vi "salRegSubEventsView.vi"(8 "error in (no error)":errorcluster, 11 "MiddlewareSALThisComponent in":refnum<class "MiddlewareSALThisComponent.lvclass">) -> (0 "error out":errorcluster, 2 "Event Registration Refnum":refnum<event-registration>, 3 "MiddlewareSALThisComponent out":refnum<class "MiddlewareSALThisComponent.lvclass">)   [LabVIEW 2016, in "MiddlewareSALThisComponent.lvclass"]
uses:
  MiddlewareSALThisComponent.lvclass
  ts_sallv_FiberSpectrograph/SALLV_FiberSpectrograph.lvlib
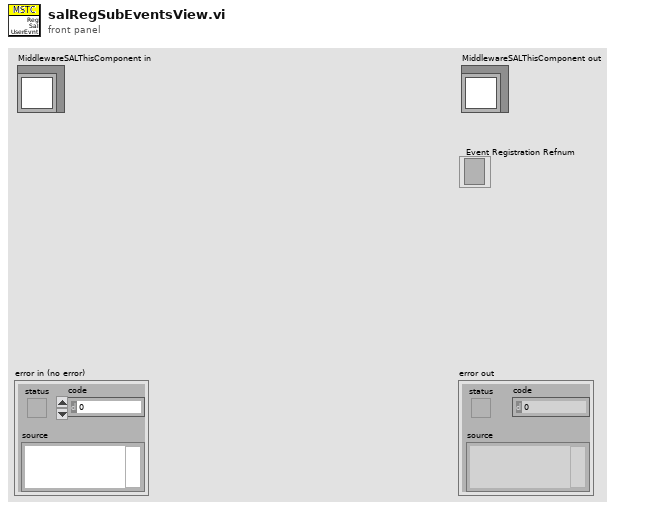
[diagram p1: front panel]
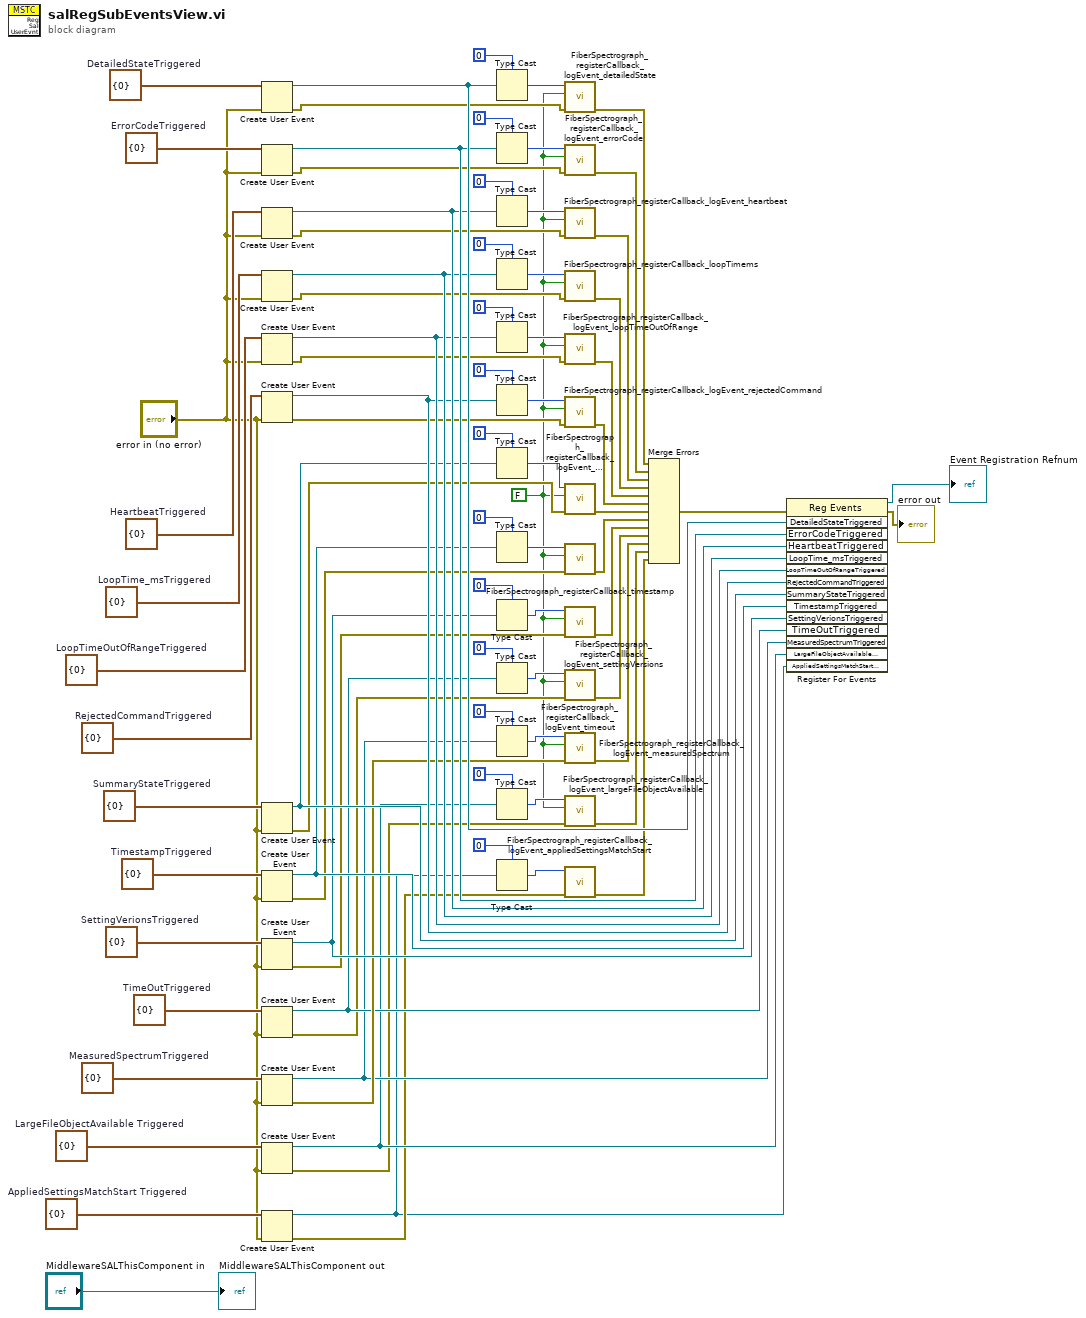
[diagram p0: block diagram]
diagram:
  w7 = cluster{"Data":i32} {"Data"=0}  # AppliedSettingsMatchStart Triggered
  w15 = cluster{"Data":i32} {"Data"=0}  # LargeFileObjectAvailable Triggered
  w18 = cluster{"Data":i32} {"Data"=0}  # TimeOutTriggered
  w26 = cluster{"Data":i32} {"Data"=0}  # MeasuredSpectrumTriggered
  w56 = cluster{"Data":i32} {"Data"=0}  # SettingVerionsTriggered
  w69 = cluster{"Data":i32} {"Data"=0}  # ErrorCodeTriggered
  w75 = cluster{"Data":i32} {"Data"=0}  # TimestampTriggered
  w74 = cluster{"Data":i32} {"Data"=0}  # SummaryStateTriggered
  w73 = cluster{"Data":i32} {"Data"=0}  # RejectedCommandTriggered
  w72 = cluster{"Data":i32} {"Data"=0}  # LoopTimeOutOfRangeTriggered
  w71 = cluster{"Data":i32} {"Data"=0}  # LoopTime_msTriggered
  w70 = cluster{"Data":i32} {"Data"=0}  # HeartbeatTriggered
  w76 = cluster{"Data":i32} {"Data"=0}  # DetailedStateTriggered
  w8 = FALSE ("skipOld")
  n1 = Create User Event(user event datatype=w76, error in="error in (no error)") -> (user event=w68:refnum<user-event>, error out=w54:errorcluster)
  n2 = Create User Event(user event datatype=w69, error in="error in (no error)") -> (user event=w67:refnum<user-event>, error out=w51:errorcluster)
  n3 = Create User Event(user event datatype=w70, error in="error in (no error)") -> (user event=w66:refnum<user-event>, error out=w48:errorcluster)
  n4 = Create User Event(user event datatype=w71, error in="error in (no error)") -> (user event=w65:refnum<user-event>, error out=w33:errorcluster)
  n5 = Create User Event(user event datatype=w72, error in="error in (no error)") -> (user event=w64:refnum<user-event>, error out=w45:errorcluster)
  n6 = Create User Event(user event datatype=w73, error in="error in (no error)") -> (user event=w63:refnum<user-event>, error out=w42:errorcluster)
  n7 = Create User Event(user event datatype=w74, error in="error in (no error)") -> (user event=w62:refnum<user-event>, error out=w39:errorcluster)
  n8 = Create User Event(user event datatype=w75, error in="error in (no error)") -> (user event=w61:refnum<user-event>, error out=w30:errorcluster)
  n9 = Create User Event(user event datatype=w56, error in="error in (no error)") -> (user event=w57:refnum<user-event>, error out=w36:errorcluster)
  n10 = Create User Event(user event datatype=w18, error in="error in (no error)") -> (user event=w21:refnum<user-event>, error out=w19:errorcluster)
  n11 = Create User Event(user event datatype=w26, error in="error in (no error)") -> (user event=w20:refnum<user-event>, error out=w22:errorcluster)
  n12 = Create User Event(user event datatype=w15, error in="error in (no error)") -> (user event=w12:refnum<user-event>, error out=w10:errorcluster)
  n13 = Create User Event(user event datatype=w7, error in="error in (no error)") -> (user event=w1:refnum<user-event>, error out=w3:errorcluster)
  n14 = Type Cast(type=0, x=w68) -> (*(type *) &x=w55:i32)
  n15 = Type Cast(type=0, x=w67) -> (*(type *) &x=w50:i32)
  n16 = Type Cast(type=0, x=w66) -> (*(type *) &x=w47:i32)
  n17 = Type Cast(type=0, x=w65) -> (*(type *) &x=w32:i32)
  n18 = Type Cast(type=0, x=w64) -> (*(type *) &x=w44:i32)
  n19 = Type Cast(type=0, x=w63) -> (*(type *) &x=w41:i32)
  n20 = Type Cast(type=0, x=w62) -> (*(type *) &x=w38:i32)
  n21 = Type Cast(type=0, x=w61) -> (*(type *) &x=w29:i32)
  n22 = Type Cast(type=0, x=w57) -> (*(type *) &x=w35:i32)
  n23 = Type Cast(type=0, x=w21) -> (*(type *) &x=w24:i32)
  n24 = Type Cast(type=0, x=w20) -> (*(type *) &x=w27:i32)
  n25 = Type Cast(type=0, x=w12) -> (*(type *) &x=w13:i32)
  n26 = Type Cast(type=0, x=w1) -> (*(type *) &x=w4:i32)
  n27 = call "FiberSpectrograph_registerCallback_logEvent_detailedState.vi"("error in (no error)"=w54, "skipOld"=w8, "handle"=w55) -> ("error out"=w53:errorcluster)  [unwired: 7 in, 1 out]
  n28 = call "FiberSpectrograph_registerCallback_logEvent_errorCode.vi"("error in (no error)"=w51, "skipOld"=w8, "handle"=w50) -> ("error out"=w52:errorcluster)  [unwired: 7 in, 1 out]
  n29 = call "FiberSpectrograph_registerCallback_logEvent_heartbeat.vi"("error in (no error)"=w48, "skipOld"=w8, "handle"=w47) -> ("error out"=w49:errorcluster)  [unwired: 7 in, 1 out]
  n30 = call "FiberSpectrograph_registerCallback_loopTimems.vi"("error in (no error)"=w33, "skipOld"=w8, "handle"=w32) -> ("error out"=w34:errorcluster)  [unwired: 7 in, 1 out]
  n31 = call "FiberSpectrograph_registerCallback_logEvent_loopTimeOutOfRange.vi"("error in (no error)"=w45, "skipOld"=w8, "handle"=w44) -> ("error out"=w46:errorcluster)  [unwired: 7 in, 1 out]
  n32 = call "FiberSpectrograph_registerCallback_logEvent_rejectedCommand.vi"("error in (no error)"=w42, "skipOld"=w8, "handle"=w41) -> ("error out"=w43:errorcluster)  [unwired: 7 in, 1 out]
  n33 = call "FiberSpectrograph_registerCallback_logEvent_summaryState.vi"("error in (no error)"=w39, "skipOld"=w8, "handle"=w38) -> ("error out"=w40:errorcluster)  [unwired: 7 in, 1 out]
  n34 = call "FiberSpectrograph_registerCallback_timestamp.vi"("error in (no error)"=w30, "skipOld"=w8, "handle"=w29) -> ("error out"=w31:errorcluster)  [unwired: 7 in, 1 out]
  n35 = call "FiberSpectrograph_registerCallback_logEvent_settingVersions.vi"("error in (no error)"=w36, "skipOld"=w8, "handle"=w35) -> ("error out"=w37:errorcluster)  [unwired: 7 in, 1 out]
  n36 = call "FiberSpectrograph_registerCallback_logEvent_timeout.vi"("error in (no error)"=w19, "skipOld"=w8, "handle"=w24) -> ("error out"=w17:errorcluster)  [unwired: 7 in, 1 out]
  n37 = call "FiberSpectrograph_registerCallback_logEvent_measuredSpectrum.vi"("error in (no error)"=w22, "skipOld"=w8, "handle"=w27) -> ("error out"=w16:errorcluster)  [unwired: 7 in, 1 out]
  n38 = call "FiberSpectrograph_registerCallback_logEvent_largeFileObjectAvailable.vi"("error in (no error)"=w10, "skipOld"=w8, "handle"=w13) -> ("error out"=w11:errorcluster)  [unwired: 7 in, 1 out]
  n39 = call "FiberSpectrograph_registerCallback_logEvent_appliedSettingsMatchStart.vi"("error in (no error)"=w3, "handle"=w4) -> ("error out"=w2:errorcluster)  [unwired: 8 in, 1 out]
  n40 = Merge Errors(w53, w52, w49, w34, w46, w43, w40, w31, w37, w17, w16, w11, w2) -> (w60:errorcluster)
  n41 = register-events(error in=w60, w68, w67, w66, w65, w64, w63, w62, w61, w57, w21, w20, w12, w1) -> (reference out=→"Event Registration Refnum":refnum<event-registration>, error out=→"error out":errorcluster)  [unwired: 1 in]
  "MiddlewareSALThisComponent out" <- "MiddlewareSALThisComponent in"
